vi "ButtonPacketSize.vi"() -> (0 "joystick packet size":u8, 1 "button packet size":u8)   [LabVIEW 2010, in "Packet Recorder.lvlib"]
uses:
  Packet Recorder.lvlib
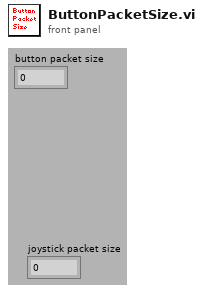
[diagram p1: front panel]
types:
  T1 = cluster{"1B1-12:2B1-12:1POV:2POV":bool[], "1LXY:RXY:2LXY:RXY":bool[]}
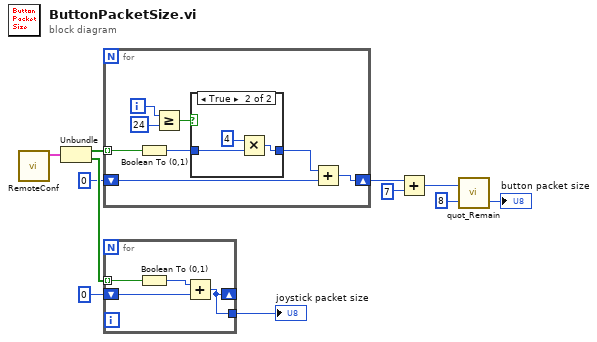
[diagram p0: block diagram]
diagram:
  n1 = call "RemoteConf.vi"() -> ("Conf"=w11:T1)  [unwired: 11 in]
  n2 = Unbundle(w11) -> ("1B1-12:2B1-12:1POV:2POV"=w10:bool[], "1LXY:RXY:2LXY:RXY"=w5:bool[])
  n3 = for {
    tunnel: w10 -> [w19] mode=indexing
    shift-right: [w12] -> w1
    shift-left: 0 -> [w16]
    i -> [w13]
    n4 = Boolean To (0,1)(Boolean=w19) -> (0, 1=w14:i16)
    n5 = Greater Or Equal?(x=w13, y=24) -> (x >= y?=w18:bool)
    n6 = case shown="True" w18 {
      tunnel: w14 -> [w20 w23]
      tunnel: [w20 w21] -> w15
      frame False {
      }
      frame True {
        n7 = Multiply(x=i16 4, y=w23) -> (x*y=w21:i16)
      }
    }
    n8 = Add(x=w15, y=w16) -> (x+y=w12:i32)
  }
  n9 = for {
    tunnel: w5 -> [w27] mode=indexing
    shift-right: [w24] -> _
    shift-left: i16 0 -> [w25]
    tunnel: [w24] -> w4
    n10 = Boolean To (0,1)(Boolean=w27) -> (0, 1=w26:i16)
    n11 = Add(x=w26, y=w25) -> (x+y=w24:i16)
  }
  "joystick packet size" <- w4
  n12 = Add(x=w1, y=7) -> (x+y=w9:i32)
  n13 = call <vilib>:"quot_Remain.vi"("y"=8, "x"=w9) -> ("floor(x/y)"=→"button packet size":i32)  [unwired: 1 out]
